vi "Empty Dictionary Datastore.vi"() -> (2 "Categories":map{string, map{string, variant}}(c390))   [LabVIEW 2021, in "Bananas.lvlib" / "Datastore.Dictionaries.lvclass"]
uses:
  Datastore.Dictionaries.lvclass
  Datastore.Dictionaries.lvclass/Datastore.Dictionaries.ctl
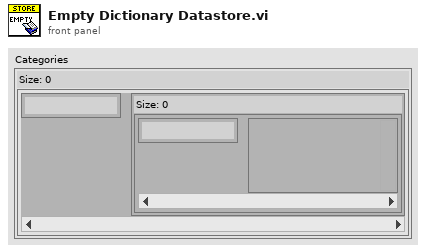
[diagram p1: front panel]
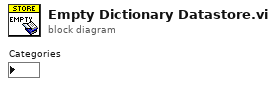
[diagram p0: block diagram]
diagram:
